vi "PDash Duplicate Event.vi"(8 "error in":errorcluster, 10 "Current Selection":T1, 11 "Project":refnum<class "Project.lvclass">) -> (0 "error out":errorcluster)   [LabVIEW 2020, in "Panther Dashboard.lvlib"]
doc: "Panther Dashboard DQMH Duplicate Event"
uses:
  Panther Dashboard.lvlib
  Class/Project/Project.lvclass
  Class/Library/Library.lvclass
  C:/GitClones/PantherLAB/PantherDashboard/src/LabVIEW/Panther Dashboard/Class/LabVIEWItem/LabVIEWItem.lvclass
  Class/VI/VI.lvclass
  Class/Library/Library.lvclass/Library.ctl
  Class/LabVIEWItem/LabVIEWItem.lvclass/LabVIEWItem.ctl
  Class/Project/Project.lvclass/Project.ctl
  <vilib>/Delacor/Delacor QMH/Libraries/_Scripting Support/Module Type--enum.ctl
  <vilib>/Delacor/Delacor QMH/Libraries/_Scripting Support/dqmh_lib_DQMH Scripting Support.lvlib
  <vilib>/Delacor/Delacor QMH/Libraries/_Scripting Support/Module Info--cluster.ctl
  Controls/Cancel.ctl
  Controls/Continue.ctl
panel:
  out "Selected Module":string caption="Current Module+ Event Selection:"
  in  "Module Description":string caption="New Module Description"
  in  "New Module Path":path
  in  "Module Name":string caption="New Event Name"
  in  "Continue":T2
  in  "Cancel":T3
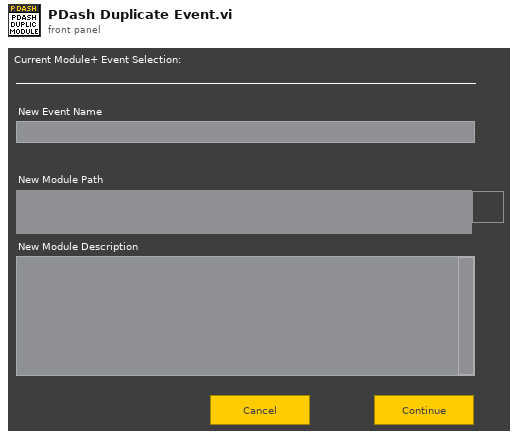
[diagram p1: front panel]
types:
  T1 = cluster{"Library":refnum<class "Library.lvclass">, "VI":refnum<class "VI.lvclass">}
  T2 = typedef "Continue.ctl" = bool
  T3 = typedef "Cancel.ctl" = bool
  T4 = typedef "dqmh_lib_DQMH Scripting Support.lvlib/Module Info--cluster.ctl" = cluster{"Name":string, "Library":refnum<vi>, "Library Owning App":refnum<vi>, "Library Owning Folder":path, "Module Type":T5, "Public API Requests Folder":refnum<vi>, "Public API Requests Arguments Folder":refnum<vi>, "Broadcasts Folder":refnum<vi>, "Broadcasts Arguments Folder":refnum<vi>, "Obtain Broadcast Events VI":refnum<vi>, "Destroy Broadcast Events VI":refnum<vi>, "Obtain Request Events VI":refnum<vi>, "Destroy Request Events VI":refnum<vi>, "Request Events Cluster CTL":refnum<vi>, "Broadcast Events Cluster CTL":refnum<vi>, "Module Timeout VI":refnum<vi>, "Module Name VI":refnum<vi>, "Status Updated VI":refnum<vi>, "Module Not Running Error Constant VI":refnum<vi>}
  T5 = typedef "dqmh_lib_DQMH Scripting Support.lvlib/Module Type--enum.ctl" = enum16{"Singleton", "Cloneable"}
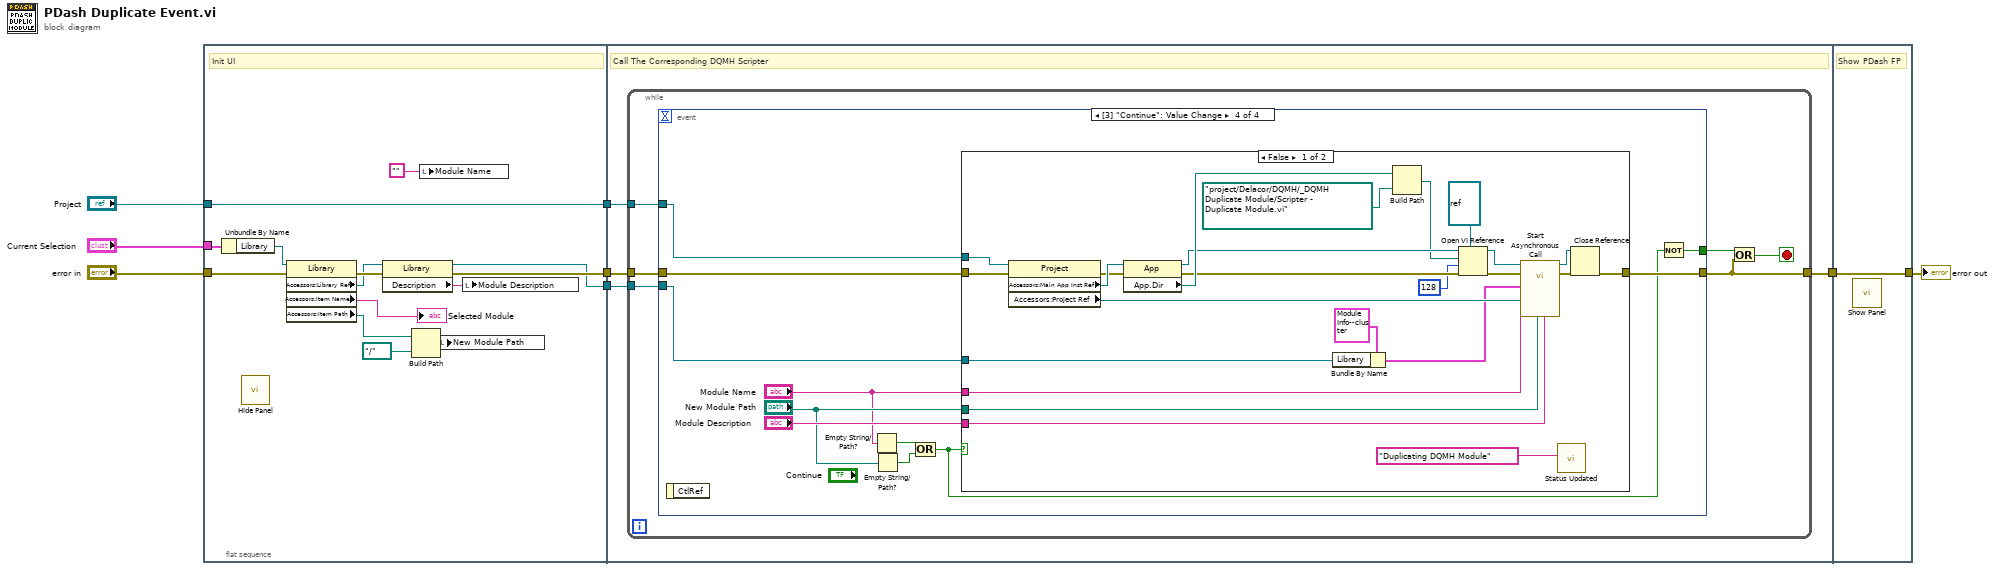
[diagram p0: block diagram]
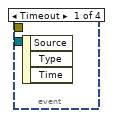
[diagram p2: hidden frame]
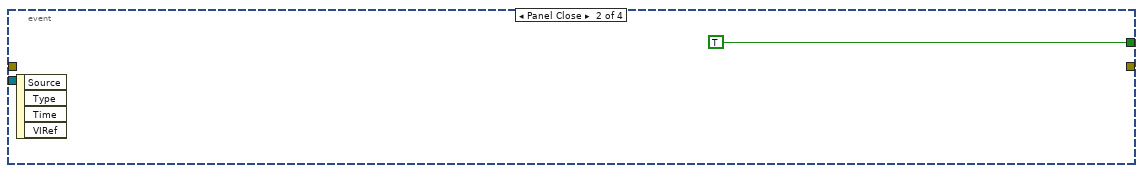
[diagram p3: hidden frame]
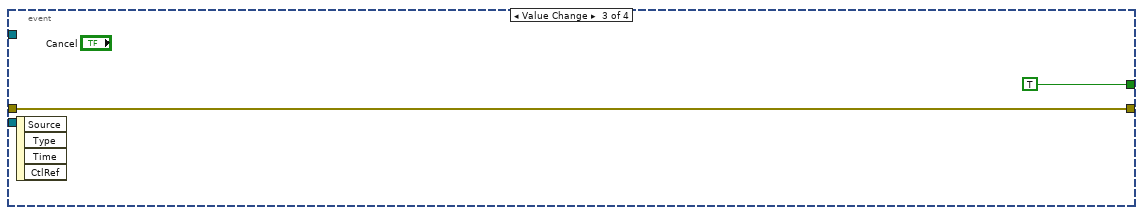
[diagram p4: hidden frame]
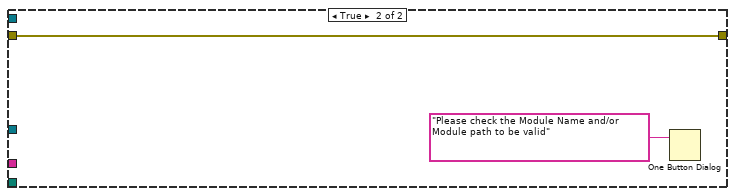
[diagram p5: hidden frame]
diagram:
  n1 = flat-sequence {
    tunnel: "Project" -> [w19]
    tunnel: [w19] -> w3
    tunnel: "error in" -> [w22]
    tunnel: [w20] -> w5
    tunnel: "Current Selection" -> [w18]
    tunnel: [w11] -> w1
    tunnel: [w26] -> w8
    tunnel: w3 -> [w24]
    tunnel: w5 -> [w25]
    tunnel: w1 -> [w23]
    tunnel: [w73] -> w7
    tunnel: w8 -> [w73]
    frame #0 {
      # "Init UI"
      n2 = Unbundle By Name(w18) -> ("Library"=w17:refnum<class "Library.lvclass">)
      n3 = call "Hide Panel.vi"() -> ()  [unwired: 11 in, 1 out]
      n4 = property class="Library"(reference=w17, error in=w22) -> (error out=w21:errorcluster, "Accessors:Library Ref"=w12:refnum<vi>, "Accessors:Item Name"=→"Selected Module":string, "Accessors:Item Path"=w14:path)  [unwired: 1 out]
      n5 = property class="Library"(reference=w12, error in=w21) -> (reference out=w11:refnum<vi>, error out=w20:errorcluster, "Description"=w10:string)
      n6 = Build Path(base path=w14, name or relative path=path "../..") -> (appended path=w16:path)
      n7 = local write "Module Name"("") -> ()
      n8 = local write "New Module Path"(w16) -> ()
      n9 = local write "Module Description"(w10) -> ()
    }
    frame #1 {
      # "Call The Corresponding DQMH Scripter"
      n10 = while {
        tunnel: [w27] -> w26
        tunnel: w24 -> [w30]
        tunnel: w25 -> [w32]
        tunnel: w23 -> [w29]
        stop <- w28 stop-if-true
        n11 = event shown="[3] \"Continue\": Value Change" {
          selector: _ -> [_ _ _ _]
          dyn-events: _ -> [_ _ _ _]
          timeout: _ -> [_ _ _ _]
          tunnel: [_ TRUE TRUE w44] -> w31
          tunnel: [_ _ w34 w37] -> w27
          tunnel: w30 -> [_ _ _ w40]
          tunnel: w32 -> [_ _ w34 w39]
          tunnel: w29 -> [_ _ _ w38]
          event Timeout {
            n12 = event-data() -> ()  [unwired: 1 in, 3 out]
          }
          event Panel Close {
            n13 = event-data() -> ()  [unwired: 1 in, 4 out]
          }
          event Value Change {
            n14 = event-data() -> ()  [unwired: 1 in, 4 out]
          }
          event Value Change {
            n15 = event-data() -> ()  [unwired: 1 in, 1 out]
            n16 = Empty String/Path?(string/path="Module Name") -> (empty?=w46:bool)
            n17 = Empty String/Path?(string/path="New Module Path") -> (empty?=w45:bool)
            n18 = Or(x=w46, y=w45) -> (x .or. y?=w36:bool)
            n19 = case shown="False" w36 {
              tunnel: "Module Description" -> [w57 _]
              tunnel: "New Module Path" -> [w56 _]
              tunnel: "Module Name" -> [w55 _]
              tunnel: w40 -> [w54 _]
              tunnel: w39 -> [w53 w71]
              tunnel: w38 -> [w51 _]
              tunnel: [w47 w71] -> w37
              frame False {
                n20 = property class="Project"(reference=w54, error in=w53) -> (error out=w61:errorcluster, "Accessors:Main App Inst Ref"=w67:refnum<vi>, "Accessors:Project Ref"=w68:refnum<vi>)  [unwired: 1 out]
                n21 = property class="App"(reference=w67, error in=w61) -> (reference out=w65:refnum<vi>, error out=w60:errorcluster, "App.Dir"=w66:path)
                n22 = Bundle By Name(cluster=T4 {"Name"="", "Library"=refnum, "Library Owning App"=refnum, "Library Owning Folder"=path "", "Module Type"=enum."Singleton", "Public API Requests Folder"=refnum, "Public API Requests Arguments Folder"=refnum, "Broadcasts Folder"=refnum, "Broadcasts Arguments Folder"=refnum, "Obtain Broadcast Events VI"=refnum, "Destroy Broadcast Events VI"=refnum, "Obtain Request Events VI"=refnum, "Destroy Request Events VI"=refnum, "Request Events Cluster CTL"=refnum, "Broadcast Events Cluster CTL"=refnum, "Module Timeout VI"=refnum, "Module Name VI"=refnum, "Status Updated VI"=refnum, "Module Not Running Error Constant VI"=refnum} ("Module Info in"), "Library"=w51) -> (w63:T4)
                n23 = Build Path(base path=w66, name or relative path=path "project/Delacor/DQMH/_DQMH Duplicate Module/Scripter - Duplicate Module.vi") -> (appended path=w62:path)
                n24 = Open VI Reference(type specifier VI Refnum (for type only)=refnum<vi> refnum, application reference (local)=w65, vi path=w62, options=128, error in (no error)=w60) -> (vi reference=w69:refnum<vi>, error out=w58:errorcluster)  [unwired: 1 in]
                n25 = call-by-ref "Start Asynchronous Call"(reference=w69, error in=w58, "Description"=w57, "Save Folder"=w56, "Project"=w68, "New Module Name"=w55, "Module Info in"=w63) -> (reference out=w64:refnum<vi>, error out=w59:errorcluster)  [unwired: 5 in, 2 out]
                n26 = call "Status Updated.vi"("Status"="Duplicating DQMH Module") -> ()  [unwired: 10 in, 1 out]
                n27 = Close Reference(reference=w64, error in (no error)=w59) -> (error out=w47:errorcluster)
              }
              frame True {
                n28 = One Button Dialog(message="Please check the Module Name and/or Module path to be valid") -> ()  [unwired: 1 in, 1 out]
              }
            }
            n29 = Not(x=w36) -> (.not. x?=w44:bool)
          }
        }
        n30 = Or(x=w31, y=w27) -> (x .or. y?=w28:bool)
      }
    }
    frame #2 {
      # "Show PDash FP"
      n31 = call "Show Panel.vi"() -> ()  [unwired: 11 in, 1 out]
    }
  }
  "error out" <- w7
